vi "Hand Type.vi"(8 "error in (no error)":errorcluster, 11 "Hand In":refnum<class "Hand with Joker.lvclass">) -> (0 "error out":errorcluster, 2 "Score":T1(ring), 3 "Hand Out":refnum<class "Hand with Joker.lvclass">)   [LabVIEW 2020, in "Hand with Joker.lvclass"]
uses:
  Hand with Joker.lvclass
  Hand with Joker.lvclass/Hand with Joker.ctl
  a02ecccc-9047-47c4-92f0-a35d10906413.vi
  3f593b3f-7ea3-4136-9a25-4e23da202726.vi
  <vilib>/Comparison/Equal/Equal Functor/Equal Functor.lvclass
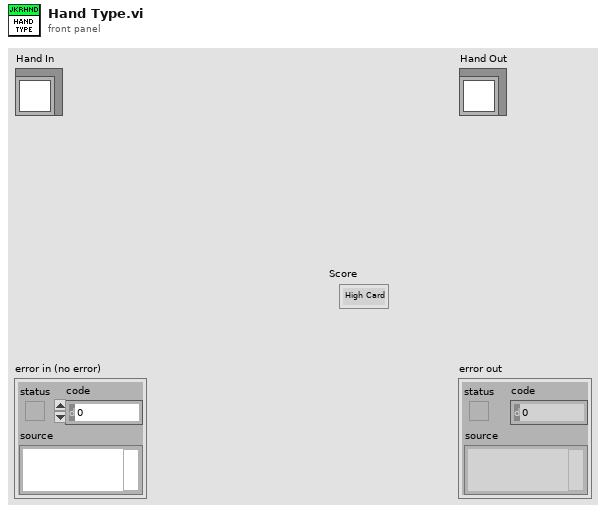
[diagram p1: front panel]
types:
  T1 = enum16{"High Card", "One Pair", "Two Pairs", "Three of a Kind", "Full House", "Four of a Kind", "Five of a Kind"}
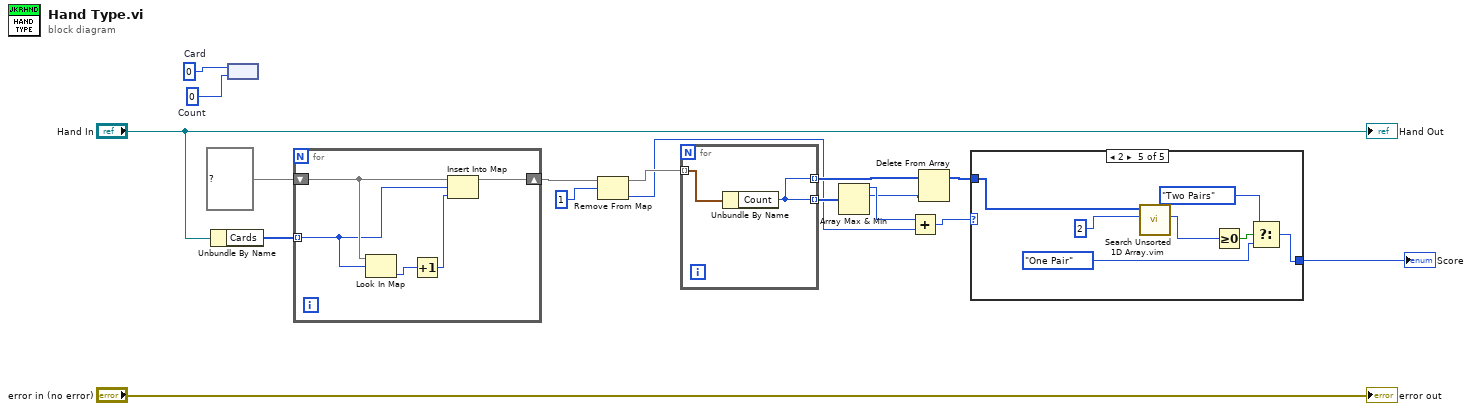
[diagram p0: block diagram]
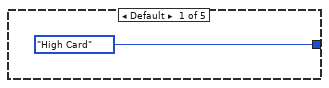
[diagram p2: hidden frame]
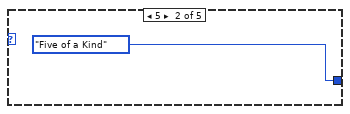
[diagram p3: hidden frame]
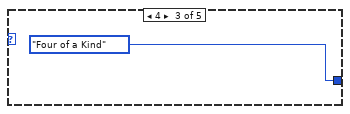
[diagram p4: hidden frame]
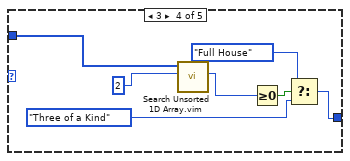
[diagram p5: hidden frame]
diagram:
  w14 = u8 0  # Count
  w15 = u8 0  # Card
  n1 = Unbundle By Name("Hand In") -> ("Cards"=w12:u8[])
  n2 = node(w15, w14) -> ()  [unwired: 1 out]
  n3 = for {
    shift-right: [w18] -> w5
    shift-left: map{u8, u8} {} ("map") -> [w22]
    tunnel: w12 -> [w21] mode=indexing
    n4 = Look In Map(map=w22, key=w21) -> (value=w20:u8)  [unwired: 1 in, 1 out]
    n5 = Increment(x=w20) -> (x+1=w19:u8)
    n6 = Insert Into Map(map in=w22, key=w21, value=w19) -> (map out=w18:map{u8, u8})  [unwired: 2 out]
  }
  n7 = Remove From Map(10:u8 1 ("key"), 11:w5) -> (1:w1:u8, 3:w4:map{u8, u8})  [unwired: 1 out]
  n8 = for {
    tunnel: [w23] -> w9 mode=indexing
    tunnel: w4 -> [w24] mode=indexing
    tunnel: [w23] -> w8 mode=indexing
    n9 = Unbundle By Name(w24) -> ("Count"=w23:u8)
  }
  n10 = Array Max & Min(array=w9) -> (max value=w11:u8, max index (indices)=w6:i32)  [unwired: 2 out]
  n11 = Add(x=w11, y=w1) -> (x+y=w2:u8)
  n12 = Delete From Array(array=w8, index=w6) -> (array with subset deleted=w7:u8[])  [unwired: 1 in, 1 out]
  n13 = case shown="2" w2 {
    tunnel: [T1."High Card" ("Score") T1."Five of a Kind" ("Score") T1."Four of a Kind" ("Score") w29 w37] -> w10
    tunnel: w7 -> [_ _ _ w34 w35]
    frame Default {
    }
    frame 5 {
    }
    frame 4 {
    }
    frame 3 {
      n14 = call "Search Unsorted 1D Array.vim"("element"=2 ("Count"), "unsorted 1D array"=w34) -> ("index of element"=w32:i32)  [unwired: 9 in]
      n15 = Greater Or Equal To 0?(x=w32) -> (x >= 0?=w31:bool)
      n16 = Select(t=T1."Full House", s=w31, f=T1."Three of a Kind" ("Score")) -> (s? t:f=w29:T1)
    }
    frame 2 {
      n17 = call "Search Unsorted 1D Array.vim"("element"=2 ("Count"), "unsorted 1D array"=w35) -> ("index of element"=w40:i32)  [unwired: 9 in]
      n18 = Greater Or Equal To 0?(x=w40) -> (x >= 0?=w39:bool)
      n19 = Select(t=T1."Two Pairs", s=w39, f=T1."One Pair" ("Score")) -> (s? t:f=w37:T1)
    }
  }
  "Score" <- w10
  "error out" <- "error in (no error)"
  "Hand Out" <- "Hand In"
